vi "Initialize MeasurementLink Session.vi"(7 "remote connection options":T2, 8 "error in":errorcluster, 9 "initialize and close session behavior":T1, 10 "session initialization parameters":T3, 11 "session factory in":refnum<class "Session Factory.lvclass">) -> (0 "error out":errorcluster, 2 "session out":variant, 3 "session factory out":refnum<class "Session Factory.lvclass">)   [LabVIEW 2021, in "NI Session Management niSwitch.lvlib" / "Session Factory.lvclass"]
doc: "Creates a new session using the provided <b>session initialization parameters</b>. If the session represents a remote session, <b>initialize and close session behavior</b> determines whether creating the local session creates a new session on the server or attaches to an existing session on the server."
uses:
  Session Factory.lvclass
  <vilib>/Plug-In SDKs/Sessions/Instrument/ISession Factory/Session Initialization Parameters.ctl
  <vilib>/Plug-In SDKs/Sessions/Instrument/ISession Factory/Remote Connection Options.ctl
  <vilib>/Plug-In SDKs/Sessions/Instrument/ISession Factory/Initialize and Close Session Behavior.ctl
  Session Factory.lvclass/Session Factory.ctl
  <vilib>/Plug-In SDKs/Sessions/Instrument/ISession Factory/ISession Factory.lvclass
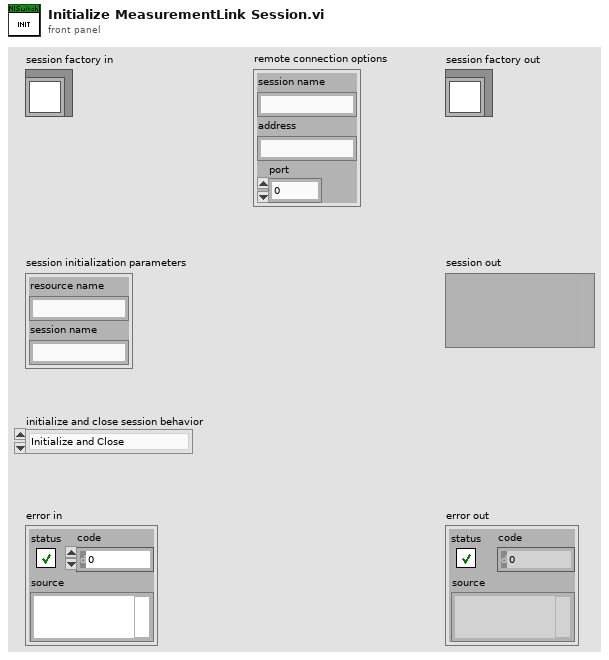
[diagram p1: front panel]
types:
  T1 = typedef "NI Session Management Instrument.lvlib/ISession Factory.lvclass/Initialize and Close Session Behavior.ctl" = enum16{"Initialize and Close", "Attach and Detach", "Initialize and Detach", "Attach and Close"}
  T2 = typedef "NI Session Management Instrument.lvlib/ISession Factory.lvclass/Remote Connection Options.ctl" = cluster{"session name":string, "address":string, "port":u32}
  T3 = typedef "NI Session Management Instrument.lvlib/ISession Factory.lvclass/Session Initialization Parameters.ctl" = cluster{"resource name":string, "session name":string}
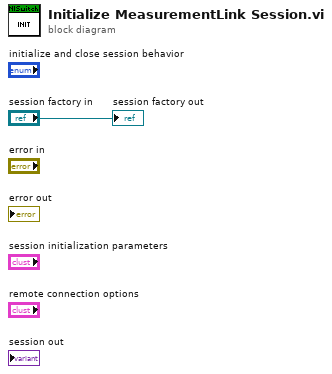
[diagram p0: block diagram]
diagram:
  "session factory out" <- "session factory in"
